vi "FTW-CodeGen-GenerateCode.vi"(0 "State In":T2 {"Width" format="%dpx"}, 5 "XRef":refnum<vi>, 7 "Terms":T1(array[cluster]), 9 "Diagram":refnum<vi>) -> (4 "State Out":T2 {"Width" format="%dpx"}, 6 "Reply":string[](array[string]), 8 "Generated Code?":bool)   [LabVIEW 2015, in "FTW-Dataflow-Burrow.xnode"]
uses:
  FTW-Dataflow-Burrow.xnode
  FTW-CodeGen-State.ctl
panel:
  # "Inputs"
  # "Outputs"
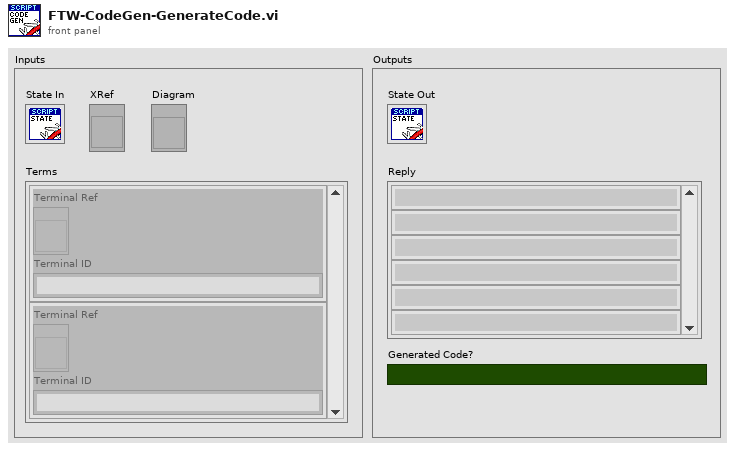
[diagram p1: front panel]
types:
  T1 = cluster{"Terminal Ref":refnum<vi>, "Terminal ID":string}[]
  T2 = typedef "FTW-Dataflow-Burrow.xnode/FTW-CodeGen-State.ctl" = cluster{"InputTerminals":cluster{"Wired?":bool, "ID":string, "DataName":string, "DataColor":u32, "Type":variant}[], "EnableTiming?":bool, "Width":i32}
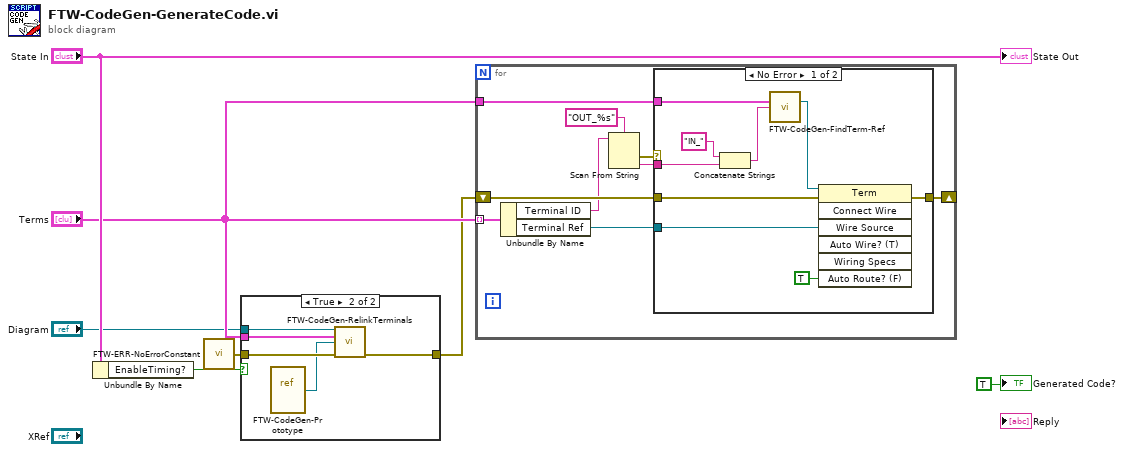
[diagram p0: block diagram]
diagram:
  n1 = Unbundle By Name("State In") -> ("EnableTiming?"=w2:bool)
  n2 = call "FTW-ERR-NoErrorConstant.vi"() -> ("no error"=w4:errorcluster)
  n3 = case shown="True" w2 {
    tunnel: "Terms" -> [_ w13]
    tunnel: w4 -> [w8 w12]
    tunnel: [w8 w11] -> w3
    tunnel: "Diagram" -> [_ w9]
    frame False {
    }
    frame True {
      n4 = vi-ref "FTW-CodeGen-Prototype.vi"() -> (w10:refnum<vi>)
      n5 = call "FTW-CodeGen-RelinkTerminals.vi"("Diagram"=w9, "Terms"=w13, "PrototypeVI"=w10, "error in"=w12) -> ("error out"=w11:errorcluster)  [unwired: 10 in, 1 out]
    }
  }
  n6 = for {
    tunnel: "Terms" -> [w22] mode=indexing
    tunnel: "Terms" -> [w15]
    shift-right: [w17] -> _
    shift-left: w3 -> [w16]
    n7 = Unbundle By Name(w22) -> ("Terminal ID"=w14:string, "Terminal Ref"=w18:refnum<vi>)
    n8 = Scan From String(format string="OUT_%s", input string=w14) -> (error out=w20:errorcluster, output 1=w19:string)  [unwired: 3 in, 2 out]
    n9 = case shown="No Error" w20 {
      tunnel: w19 -> [w30 _]
      tunnel: w18 -> [w23 _]
      tunnel: [w29 w32] -> w17
      tunnel: w16 -> [w25 w32]
      tunnel: w15 -> [w27 _]
      frame No Error {
        n10 = Concatenate Strings("IN_" ("string"), w30) -> (w28:string)
        n11 = call "FTW-CodeGen-FindTerm-Ref.vi"("Terms"=w27, "Terminal ID"=w28) -> ("Terminal Ref"=w26:refnum<vi>)  [unwired: 12 in, 1 out]
        n12 = invoke class="Term" method="Connect Wire"(reference=w26, error in=w25, "Wire Source"=w23, "Auto Route? (F)"=TRUE) -> (error out=w29:errorcluster)  [unwired: 3 in, 6 out]
      }
      frame Error {
      }
    }
  }
  "State Out" <- "State In"
  "Generated Code?" <- TRUE ("Generated Code?")
